vi "Get_LinearAcceleration.vi"(5 "Device Number":T1, 7 "Update":bool) -> (2 "Linear Acceleration":T2)   [LabVIEW 2016]
doc: "This navX VI returns the linear acceleration from the navX."
uses:
  TypeDefs/Z900_navX_DeviceRegisters.ctl
  navX Library v2.lvlib
  TypeDefs/FRIC_navX_DeviceNumbersTypeDef.ctl
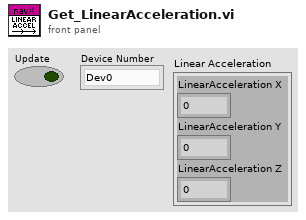
[diagram p1: front panel]
types:
  T1 = typedef "FRIC_navX_DeviceNumbersTypeDef.ctl" = enum16{"Dev0", "Dev1", "Dev2", "Dev3"}
  T2 = cluster{"LinearAcceleration X":dbl, "LinearAcceleration Y":dbl, "LinearAcceleration Z":dbl}
  T3 = typedef "navX Library v2.lvlib/Z900_navX_DeviceRegisters.ctl" = u8
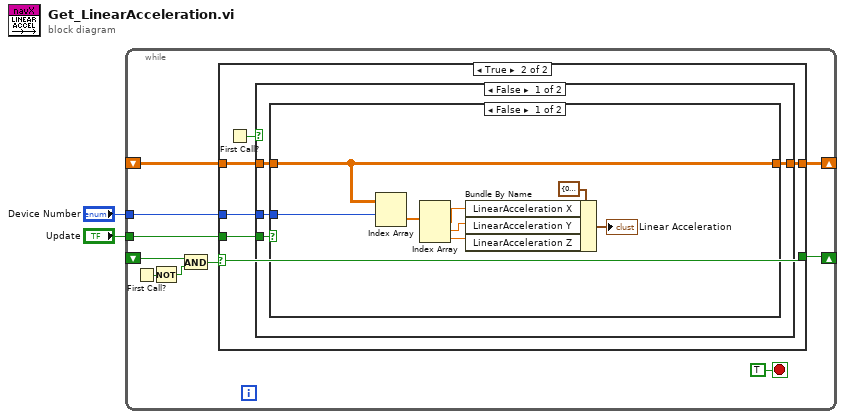
[diagram p0: block diagram]
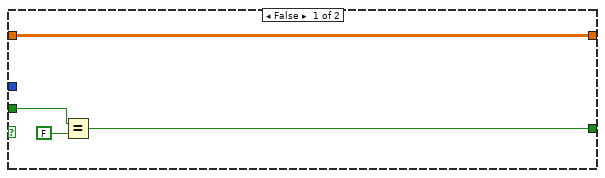
[diagram p2: hidden frame]
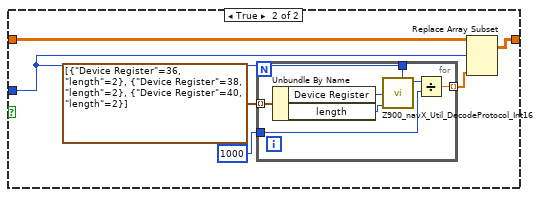
[diagram p3: hidden frame]
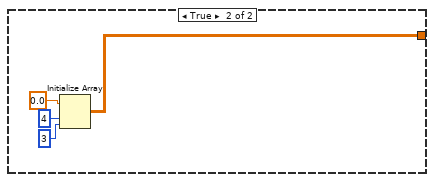
[diagram p4: hidden frame]
diagram:
  n1 = while {
    shift-right: [w12] -> _
    shift-left: _ -> [w9]
    tunnel: "Update" -> [w10]
    tunnel: "Device Number" -> [w8]
    shift-right: [w3] -> _
    shift-left: _ -> [w5]
    stop <- TRUE stop-if-true
    n2 = First Call?() -> (First Call?: T/F=w7:bool)
    n3 = Not(x=w7) -> (.not. x?=w6:bool)
    n4 = And(x=w5, y=w6) -> (x .and. y?=w4:bool)
    n5 = case shown="True" w4 {
      selector: w4 -> [_ w17]
      tunnel: [w13 w22] -> w12
      tunnel: w10 -> [w15 w21]
      tunnel: w9 -> [w13 w20]
      tunnel: w8 -> [_ w18]
      tunnel: [w14 w17] -> w3
      frame False {
        n6 = Equal?(x=w15, y=FALSE) -> (x = y?=w14:bool)
      }
      frame True {
        n7 = First Call?() -> (First Call?: T/F=w19:bool)
        n8 = case shown="False" w19 {
          tunnel: [w26 w50] -> w22
          tunnel: w21 -> [w23 _]
          tunnel: w20 -> [w25 _]
          tunnel: w18 -> [w24 _]
          frame False {
            n9 = case shown="False" w23 {
              tunnel: [w28 w38] -> w26
              tunnel: w25 -> [w28 w40]
              tunnel: w24 -> [w27 w39]
              frame False {
                n10 = Index Array(array=w28, index (row)=w27) -> (element=w34:dbl[])  [unwired: 1 in]
                n11 = Index Array(array=w34) -> (element #1=w31:dbl, element #2=w32:dbl, element #3=w33:dbl)  [unwired: 3 in]
                n12 = Bundle By Name(cluster=T2 {"LinearAcceleration X"=0.0, "LinearAcceleration Y"=0.0, "LinearAcceleration Z"=0.0} ("Linear Acceleration"), "LinearAcceleration X"=w31, "LinearAcceleration Y"=w32, "LinearAcceleration Z"=w33) -> (→"Linear Acceleration":T2)
              }
              frame True {
                n13 = for {
                  tunnel: cluster{"Device Register":T3, "length":i32}[] [{"Device Register"=36, "length"=2}, {"Device Register"=38, "length"=2}, {"Device Register"=40, "length"=2}] ("Array") -> [w45] mode=indexing
                  tunnel: w39 -> [w44]
                  tunnel: 1000 ("y") -> [w42]
                  tunnel: [w41] -> w35 mode=indexing
                  n14 = Unbundle By Name(w45) -> ("Device Register"=w47:T3, "length"=w46:i32)
                  n15 = call "Z900_navX_Util_DecodeProtocol_Int16.vi"("Device Number"=w44, "length"=w46, "Device Register"=w47) -> ("Value"=w43:i16)  [unwired: 8 in]
                  n16 = Divide(x=w43, y=w42) -> (x/y=w41:dbl)
                }
                n17 = Replace Array Subset(array=w40, new element=w35, index (row)=w39) -> (w38:dbl[][])  [unwired: 1 in]
              }
            }
          }
          frame True {
            n18 = Initialize Array(0.0, 4 ("dimension size"), 3 ("dimension size")) -> (w50:dbl[][])
          }
        }
      }
    }
  }
